vi "Auto_Inflate.vi"(9 "Data In":dbl[](array[numeric]), 11 "Item_Refnums_Array":T1[](array[typedef])) -> (1 "Data Out":dbl[](array[numeric]), 3 "Item_Refnums_Array Out":T1[](array[typedef]), 4 "Inflate/Deflate?":bool)   [LabVIEW 2011, in "Root_XControl.xctl"]
uses:
  Root_XControl.xctl
  Controls/References/Item_Refnums.ctl
  Controls/References/Item_Command_Refnum.ctl
  Controls/Item_Command_Enum.ctl
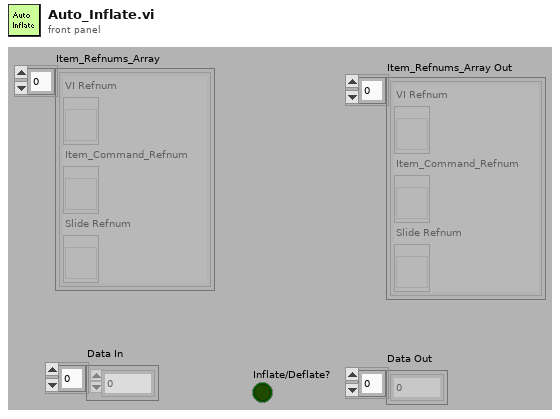
[diagram p1: front panel]
types:
  T1 = typedef "Item_Refnums.ctl" = cluster{"VI Refnum":refnum<vi>, "Item_Command_Refnum":T2, "Slide Refnum":refnum<vi>}
  T2 = typedef "Item_Command_Refnum.ctl" = refnum<vi>
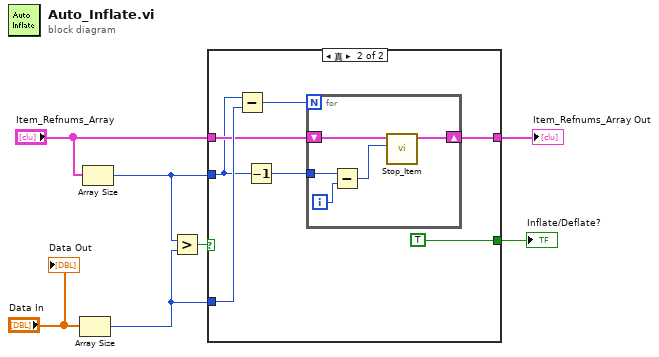
[diagram p0: block diagram]
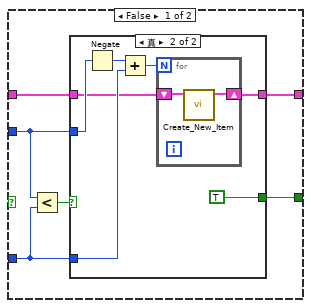
[diagram p2: hidden frame]
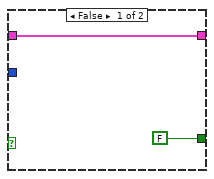
[diagram p3: hidden frame]
diagram:
  n1 = Array Size(array="Data In") -> (size(s)=w4:i32)
  n2 = Array Size(array="Item_Refnums_Array") -> (size(s)=w6:i32)
  n3 = Greater?(x=w6, y=w4) -> (0:w5:bool)
  n4 = case shown="真" w5 {
    tunnel: w6 -> [w12 w28]
    tunnel: w4 -> [w11 w31]
    tunnel: "Item_Refnums_Array" -> [w10 w29]
    tunnel: [w9 w26] -> w2
    tunnel: [w8 TRUE] -> w1
    frame False {
      n5 = Less?(x=w12, y=w11) -> (x < y?=w13:bool)
      n6 = case shown="真" w13 {
        tunnel: w12 -> [_ w22]
        tunnel: w11 -> [_ w20]
        tunnel: w10 -> [w15 w18]
        tunnel: [w15 w17] -> w9
        tunnel: [FALSE TRUE] -> w8
        frame False {
        }
        frame True {
          n7 = Negate(x=w22) -> (-x=w21:i32)
          n8 = Add(x=w21, y=w20) -> (x+y=w19:i32)
          n9 = for {
            N: w19 -> [_]
            shift-right: [w23] -> w17
            shift-left: w18 -> [w24]
            n10 = call "Create_New_Item.vi"("Item_Refnums_Array In"=w24) -> ("Item_Refnums_Array Out"=w23:T1[])  [unwired: 9 in, 1 out]
          }
        }
      }
    }
    frame True {
      n11 = Subtract(x=w28, y=w31) -> (x-y=w30:i32)
      n12 = Decrement(x=w28) -> (x-1=w27:i32)
      n13 = for {
        N: w30 -> [_]
        tunnel: w27 -> [w34]
        shift-right: [w35] -> w26
        shift-left: w29 -> [w36]
        i -> [w33]
        n14 = Subtract(x=w34, y=w33) -> (x-y=w32:i32)
        n15 = call "Stop_Item.vi"("Index"=w32, "Item_Refnums_Array"=w36) -> ("Item_Refnums_Array Out"=w35:T1[])  [unwired: 8 in, 1 out]
      }
    }
  }
  "Item_Refnums_Array Out" <- w2
  "Inflate/Deflate?" <- w1
  "Data Out" <- "Data In"
